vi "ppm oder Prozent in ppm umrechnen.vi"(9 "Einheit":string, 11 "Werteingang":string) -> (3 "Wertausgang":string)   [LabVIEW 2020, in "Linearisierung v2.lvlib" / "Gasteiler.lvlib"]
uses:
  Gasteiler.lvlib
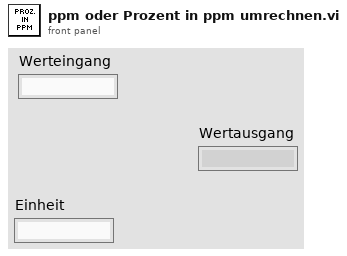
[diagram p1: front panel]
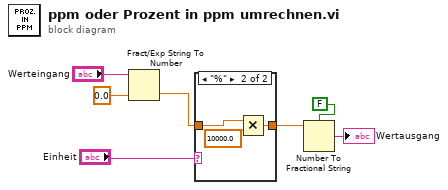
[diagram p0: block diagram]
diagram:
  n1 = Fract/Exp String To Number(string="Werteingang", default (0 dbl)=sgl 0.0 ("x")) -> (number=w4:sgl)  [unwired: 2 in, 1 out]
  n2 = case shown="\"%\"" "Einheit" {
    tunnel: [w8 w10] -> w3
    tunnel: w4 -> [w8 w9]
    frame "ppm", Default {
      # "ppm"
    }
    frame "%" {
      n3 = Multiply(x=w9, y=sgl 10000.0 ("x")) -> (x*y=w10:sgl)
    }
  }
  n4 = Number To Fractional String(use system decimal point (T)=FALSE ("Systemdezimalzeichen verwenden (T)"), number=w3) -> (F-format string=→"Wertausgang":string)  [unwired: 2 in]
